vi "Read Table Data.vi"(8 "error in":errorcluster, 11 "Table Ref in":refnum<vi>) -> (0 "error out":errorcluster, 1 "Value":string[][](array[string]), 2 "Interpret As Unicode":bool, 3 "Table Ref out":refnum<vi>)   [LabVIEW 2020, in "G-Unicode.lvlib"]
uses:
  G-Unicode.lvlib
  Unicode/SubVIs/Byte Order Marks.vi
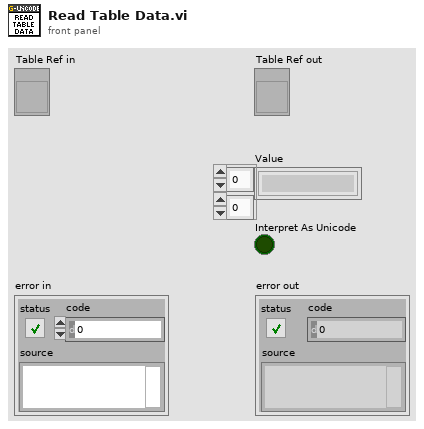
[diagram p1: front panel]
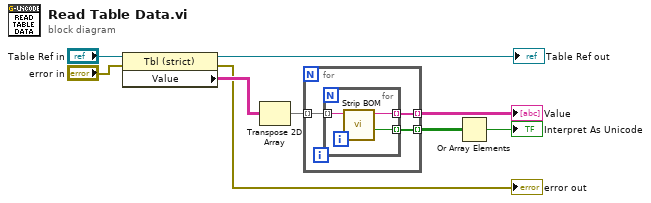
[diagram p0: block diagram]
diagram:
  n1 = property class="Tbl (strict)"(reference="Table Ref in", error in="error in") -> (reference out=→"Table Ref out":refnum<vi>, error out=→"error out":errorcluster, "Value"=w9:string[][])
  n2 = Transpose 2D Array(2D array=w9) -> (transposed array=w8:string[][])
  n3 = for {
    tunnel: w8 -> [w12] mode=indexing
    tunnel: [w11] -> w3 mode=indexing
    tunnel: [w10] -> w7 mode=indexing
    n4 = for {
      tunnel: w12 -> [w15] mode=indexing
      tunnel: [w14] -> w11 mode=indexing
      tunnel: [w13] -> w10 mode=indexing
      n5 = call "Strip BOM.vi"("String"=w15) -> ("BOM Found"=w13:bool, "String without BOM"=w14:string)  [unwired: 8 in, 1 out]
    }
  }
  "Value" <- w3
  n6 = Or Array Elements(Boolean array=w7) -> (logical OR=→"Interpret As Unicode":bool)
